vi "Constants.vi"   [LabVIEW 2027, in "Memory Manager.lvlib"]
uses:
  Memory Manager.lvlib
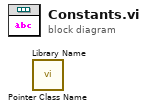
[diagram p0: block diagram]
diagram:
  n1 = call "Pointer Class Name.vi"() -> ()  [unwired: 11 in, 1 out]
  n2 = call "Library Name.vi"() -> ()  [unwired: 11 in, 1 out]
